vi "V&V Basic Receive.vi"() -> ()   [LabVIEW 2012, in "UART_Host_Driver.lvlib" / "UART Driver.lvclass"]
doc: "This example calls the UART Initialize, UART Configure Port, UART Execute Command, and a UART Close."
uses:
  UART Driver.lvclass
  Typedefs/Configuration Parameters.ctl
  FPGA/UART/StopBits.ctl
  FPGA/UART/Parity.ctl
  <vilib>/Instr/_visa.llb/VISA Configure Serial Port (Instr).vi
  FPGA/UART/UART_Firmware.lvlib
  UART_Host_Driver.lvlib
panel:
  out "Number of Read Errors":i32
  out "Number of Reads Executed":i32
  out "Receive Data":string
  in  "stop":bool
  in  "Configuration Parameters":T1={"Baud"=115200, "Character Length"=8, "Stop Bits"=enum."1.0", "Parity"=enum."None", "Character Spacing (ticks)"=0}
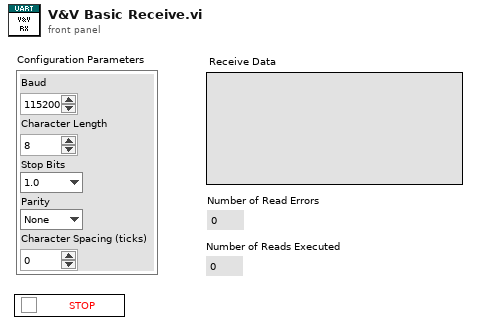
[diagram p1: front panel]
types:
  T1 = typedef "UART_Host_Driver.lvlib/Configuration Parameters.ctl" = cluster{"Baud":u32, "Character Length":u8, "Stop Bits":T2, "Parity":T3, "Character Spacing (ticks)":u32}
  T2 = typedef "UART_Firmware.lvlib/StopBits.ctl" = enum8{"1.0", "1.5", "2.0"}
  T3 = typedef "UART_Firmware.lvlib/Parity.ctl" = enum8{"None", "Even", "Odd"}
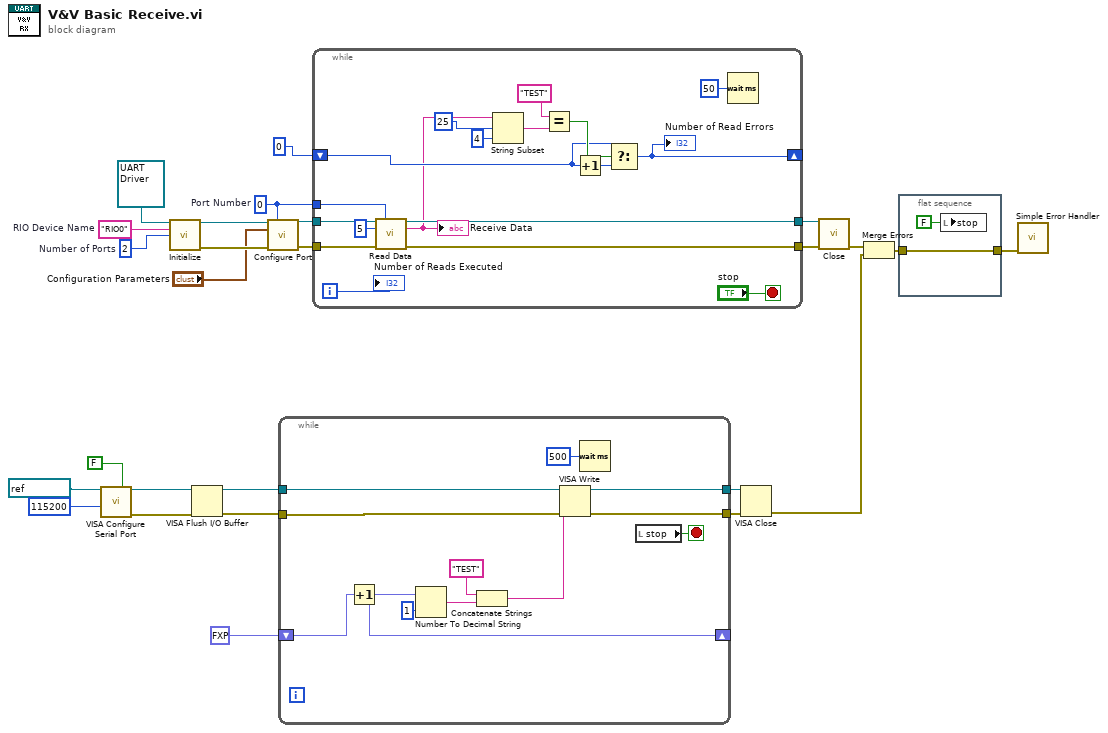
[diagram p0: block diagram]
diagram:
  w18 = u8 0  # Port Number
  w22 = u8 2  # Number of Ports
  w23 = "RIO0"  # RIO Device Name
  n1 = call-poly "VISA Configure Serial Port"("VISA resource name"=refnum<visa-resource-name> "COM1", "Enable Termination\nChar (T)"=FALSE ("Enable Termination\nChar (T)"), "baud rate (9600)"=u32 115200) -> ("VISA resource name out"=w10:refnum<visa-resource-name>, "error out"=w9:errorcluster)  [unwired: 11 in]
  n2 = call-dynamic "Initialize.vi"("UART Driver in"=refnum<class "UART Driver.lvclass"> refnum, "RIO Device Name"=w23, "Number of UART Controllers"=w22) -> ("UART Driver out"=w26:refnum<class "UART Driver.lvclass">, "error out"=w25:errorcluster)  [unwired: 11 in]
  n3 = VISA Flush I/O Buffer(VISA resource name=w10, error in (no error)=w9) -> (VISA resource name out=w7:refnum<visa-resource-name>, error out=w8:errorcluster)  [unwired: 1 in]
  n4 = call-dynamic "Configure Port.vi"("UART Driver in"=w26, "Controller Number"=w18, "Configuration Parameters"="Configuration Parameters", "error in"=w25) -> ("UART Driver out"=w20:refnum<class "UART Driver.lvclass">, "error out"=w19:errorcluster)  [unwired: 10 in]
  n5 = while {
    tunnel: w8 -> [w37]
    tunnel: w7 -> [w38]
    tunnel: [w36] -> w11
    tunnel: [w35] -> w12
    shift-right: [w29] -> _
    shift-left: fxp<+,3,3> 0.0 -> [w30]
    stop <- w33 stop-if-true
    n6 = Increment(x=w30) -> (x+1=w29:fxp<+,3,3>)
    n7 = Number To Decimal String(number=w29, width (-)=i16 1) -> (decimal integer string=w32:string)
    n8 = Concatenate Strings("TEST" ("x"), w32) -> (w27:string)
    n9 = VISA Write(VISA resource name=w38, write buffer=w27, error in (no error)=w37) -> (VISA resource name out=w35:refnum<visa-resource-name>, error out=w36:errorcluster)  [unwired: 1 out]
    n10 = Wait (ms)(milliseconds to wait=u32 500) -> ()  [unwired: 1 out]
    n11 = local read "stop"() -> (w33:bool)
  }
  n12 = while {
    tunnel: w20 -> [w56]
    tunnel: w19 -> [w55]
    tunnel: w18 -> [w54]
    tunnel: [w53] -> w17
    tunnel: [w52] -> w16
    shift-right: [w40] -> _
    shift-left: 0 -> [w43]
    i -> [w41]
    stop <- "stop" stop-if-true
    n13 = call-dynamic "Read Data.vi"("UART Driver in"=w56, "Port Number"=w54, "Rx byte count"=u32 5, "error in"=w55) -> ("UART Driver out"=w52:refnum<class "UART Driver.lvclass">, "Receive Data"=w42:string, "error out"=w53:errorcluster)  [unwired: 9 in]
    "Receive Data" <- w42
    n14 = String Subset(string=w42, offset (0)=25 ("length (rest)"), length (rest)=4 ("length (rest)")) -> (substring=w47:string)
    n15 = Equal?(x="TEST", y=w47) -> (x = y?=w45:bool)
    n16 = Increment(x=w43) -> (x+1=w44:i32)
    n17 = Select(t=w43, s=w45, f=w44) -> (s? t:f=w40:i32)
    "Number of Read Errors" <- w40
    n18 = Wait (ms)(milliseconds to wait=u32 50) -> ()  [unwired: 1 out]
    "Number of Reads Executed" <- w41
  }
  n19 = VISA Close(VISA resource name=w12, error in (no error)=w11) -> (error out=w3:errorcluster)
  n20 = call-dynamic "Close.vi"("UART Driver in"=w16, "error in"=w17) -> ("error out"=w4:errorcluster)  [unwired: 13 in]
  n21 = Merge Errors(w4, w3) -> (w2:errorcluster)
  n22 = flat-sequence {
    tunnel: w2 -> [w58]
    tunnel: [w58] -> w1
    frame #0 {
      n23 = local write "stop"(FALSE ("stop")) -> ()
    }
  }
  n24 = call <vilib>:"Simple Error Handler.vi"("error in (no error)"=w1) -> ()  [unwired: 4 in, 5 out]
